vi "HT3_Read.vi"(7 "Start From Top":bool, 8 "error in":errorcluster, 10 "Data count":i32=1, 11 "refnum in":refnum<file>) -> (0 "error out":errorcluster, 2 "Data out":u32[](array[numeric]), 3 "refnum out":refnum<file>, 4 "EOF?":bool)   [LabVIEW 2011]
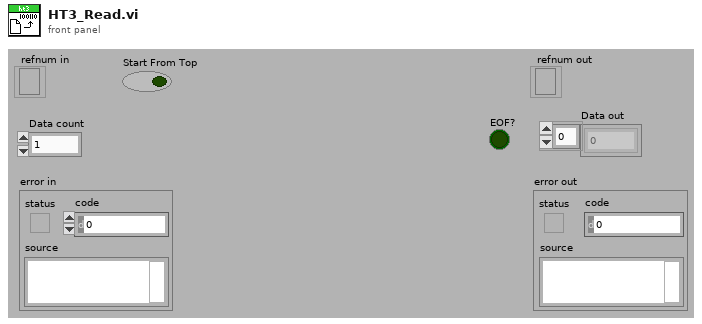
[diagram p1: front panel]
types:
  T1 = enum16{"big-endian, network order", "native, host order", "little-endian"}
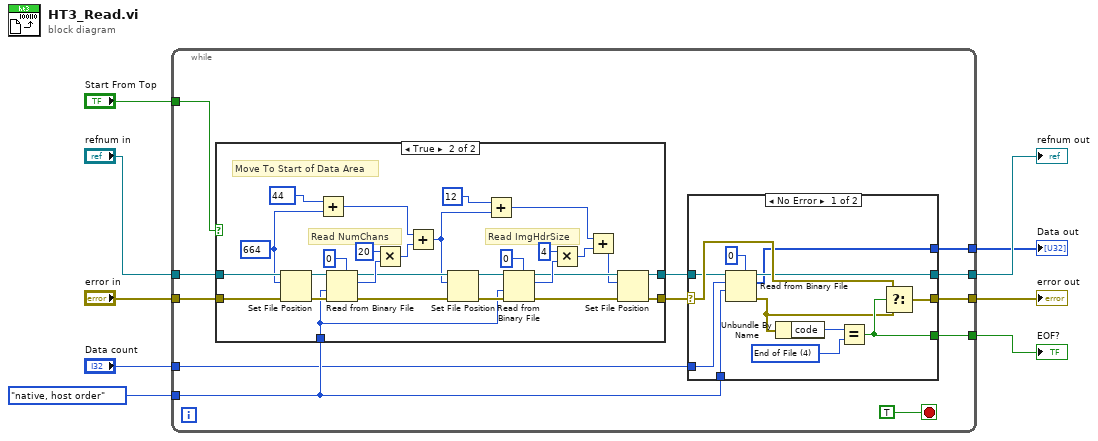
[diagram p0: block diagram]
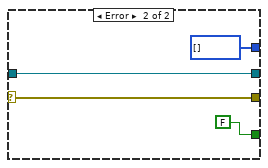
[diagram p2: hidden frame]
diagram:
  n1 = while {
    tunnel: "error in" -> [w20]
    tunnel: "refnum in" -> [w19]
    tunnel: T1."native, host order" ("byte order (0:big-endian, network order)") -> [w17]
    tunnel: "Start From Top" -> [w18]
    tunnel: [w15] -> w5
    tunnel: [w14] -> w4
    tunnel: "Data count" -> [w12]
    tunnel: [w11] -> w2
    tunnel: [w10] -> w1
    stop <- TRUE stop-if-true
    n2 = case shown="True" w18 {
      tunnel: w20 -> [w39 w67]
      tunnel: w19 -> [w38 w66]
      tunnel: w17 -> [_ w49]
      tunnel: [w39 w47] -> w16
      tunnel: [w38 w46] -> w13
      frame False {
      }
      frame True {
        w57 = i64 664 ("offset (in bytes) (0)")
        # "Read ImgHdrSize"
        # "Read NumChans"
        # "Move To Start of Data Area"
        n3 = Set File Position(offset (in bytes) (0)=w57, refnum=w66, error in=w67) -> (refnum out=w63:refnum<file>, error out=w64:errorcluster)  [unwired: 1 out]
        n4 = Add(x=i64 44 ("offset (in bytes) (0)"), y=w57) -> (x+y=w55:i64)
        n5 = Read from Binary File(5:0, 8:w64, 9:w49, 11:w63) -> (0:w59:errorcluster, 2:w62:i32, 3:w58:refnum<file>)  [unwired: 3 out]
        n6 = Multiply(x=20, y=w62) -> (x*y=w60:i32)
        n7 = Add(x=w55, y=w60) -> (x+y=w42:i64)
        n8 = Set File Position(offset (in bytes) (0)=w42, refnum=w58, error in=w59) -> (refnum out=w50:refnum<file>, error out=w51:errorcluster)  [unwired: 1 out]
        n9 = Add(x=i64 12 ("offset (in bytes) (0)"), y=w42) -> (x+y=w41:i64)
        n10 = Read from Binary File(5:0, 8:w51, 9:w49, 11:w50) -> (0:w48:errorcluster, 2:w53:i32, 3:w45:refnum<file>)  [unwired: 3 out]
        n11 = Multiply(x=4, y=w53) -> (x*y=w44:i32)
        n12 = Add(x=w41, y=w44) -> (x+y=w43:i64)
        n13 = Set File Position(offset (in bytes) (0)=w43, refnum=w45, error in=w48) -> (refnum out=w46:refnum<file>, error out=w47:errorcluster)  [unwired: 1 out]
      }
    }
    n14 = case shown="No Error" w16 {
      selector: w16 -> [w28 w37]
      tunnel: w17 -> [w33 _]
      tunnel: [w26 w37] -> w14
      tunnel: [w29 FALSE] -> w15
      tunnel: w13 -> [w25 w35]
      tunnel: [w24 w35] -> w11
      tunnel: w12 -> [w23 _]
      tunnel: [w22 u32[] []] -> w10
      frame No Error {
        w31 = 4 items=["No Error", "Manager Argument Error", "Memory Full", "Out of Zone", "End of File", "File Already Open", "Generic File IO Error", "File Not Found", "File Permission Error", "Disk Full", "Duplicate Path", "Too Many Files Open", "Not Enabled", "Resource File Not Found", "Cannot Add Resource", "Resource Not Found", "Image Not Found", "Image Memory Error", "Pen Does Not Exist", "Config Bad Type", "Config Token Not Found", "Config Parse Error", "Config Memory Error", "Bad External Code Format", "Bad External Code Offset", "External Code Not Present", "Null Window", "Destroy Window Mixup", "Null Menu", "Print Aborted", "Bad Print Record", "Print Driver Error", "Windows Error During Print", "Memory Error During Print", "Print Dialog Error", "Generic Print Error", "Invalid Device Refnum", "Device Not Found", "Device Parameter Error", "Device Unit Error", "Can't Open Device", "Device Call Aborted", "Generic Error", "Cancelled By User", "Object ID Too Low", "Object ID Too High", "Object Not In Heap", "Unknown Heap", "Bad DefProc ID", "DefProc Not In Table", "Message Out Of Range", "Null Method", "Unknown Message", "Manager Call Not Supported"]
        n15 = Read from Binary File(5:u32 0, 9:w33, 10:w23, 11:w25) -> (0:w27:errorcluster, 2:w22:u32[], 3:w24:refnum<file>)  [unwired: 1 in, 2 out]
        n16 = Unbundle By Name(w27) -> ("code"=w30:i32)
        n17 = Equal?(x=w30, y=w31) -> (x = y?=w29:bool)
        n18 = Select(t=w28, s=w29, f=w27) -> (s? t:f=w26:errorcluster)
      }
      frame Error {
      }
    }
  }
  "refnum out" <- w2
  "error out" <- w4
  "EOF?" <- w5
  "Data out" <- w1
